vi "array2Mem_32bit_1to12_pipe.vi"(6 "Address (Max = 255)":u8=24, 10 "array_in":T1=[0.0, 0.0, 0.0, 0.0, 0.0, 0.0, 0.0, 0.0, 0.0, 0.0, 0.0, 0.0]) -> ()   [LabVIEW 2017]
uses:
  ziyi_pipe.ctl
  x_qp_scalar.ctl
  <vilib>/rvi/DataTransferAndStorage/Container/Common/niFpgaContainerExecOnDevCompGetState.vi
  <vilib>/rvi/Emulation/niFpgaEmulationIsFPGAContextNoSignature.vi
  <vilib>/rvi/DataTransferAndStorage/Container/Common/niFpgaContainerGetUniqueNameForEmu.vi
  <vilib>/rvi/Emulation/niFpgaProcessEmulError.vi
  <vilib>/rvi/Emulation/niFpgaSctlEmulationGetInTimedLoop.vi
  <vilib>/rvi/errors/nirviReportUnexpectedCaseInternalError (U32).vi
  <vilib>/rvi/Memory/Memory_Emulation/niFpgaMemoryEmulationCacheClearOnFirstRun.vi
  <vilib>/rvi/Memory/Memory_Emulation/nirvimemoryEmulationManagerCache_MakeExclusive.vi
  <vilib>/rvi/Memory/Memory_Emulation/niFpgaMemoryEmulationValidateCache.vi
  <vilib>/rvi/Memory/Memory_Emulation/nirvimemoryEmulationManagerCache_InsertValue.vi
  <vilib>/Utility/error.llb/Clear Errors.vi
  <vilib>/rvi/Memory/Memory_Emulation/nirvimemoryEmulationManagerCache_ReleaseExclusive.vi
  <vilib>/rvi/Memory/Memory_Emulation/nirvimemoryEmulationManagerCache_GetValue.vi
  <vilib>/rvi/Memory/Memory_Emulation/nirvimemoryEmulationManagerCache_SetValue.vi
  <vilib>/rvi/Emulation/niFpgaSctlEmulationResourceMgr.vi
  <vilib>/rvi/DataTransferAndStorage/Container/XNode/niFpgaContainer.xnode
  <vilib>/rvi/Memory/Memory_Emulation/niFpgaMemoryEmulationRefIn.vi
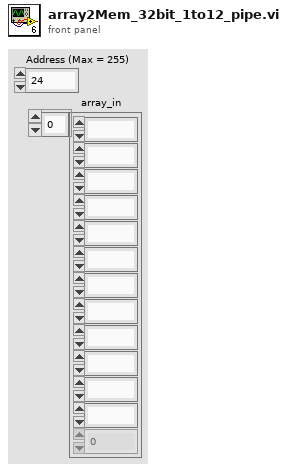
[diagram p1: front panel]
types:
  T1 = typedef "ziyi_pipe.ctl" = T2[]
  T2 = typedef "x_qp_scalar.ctl" = fxp<+/-,32,6>
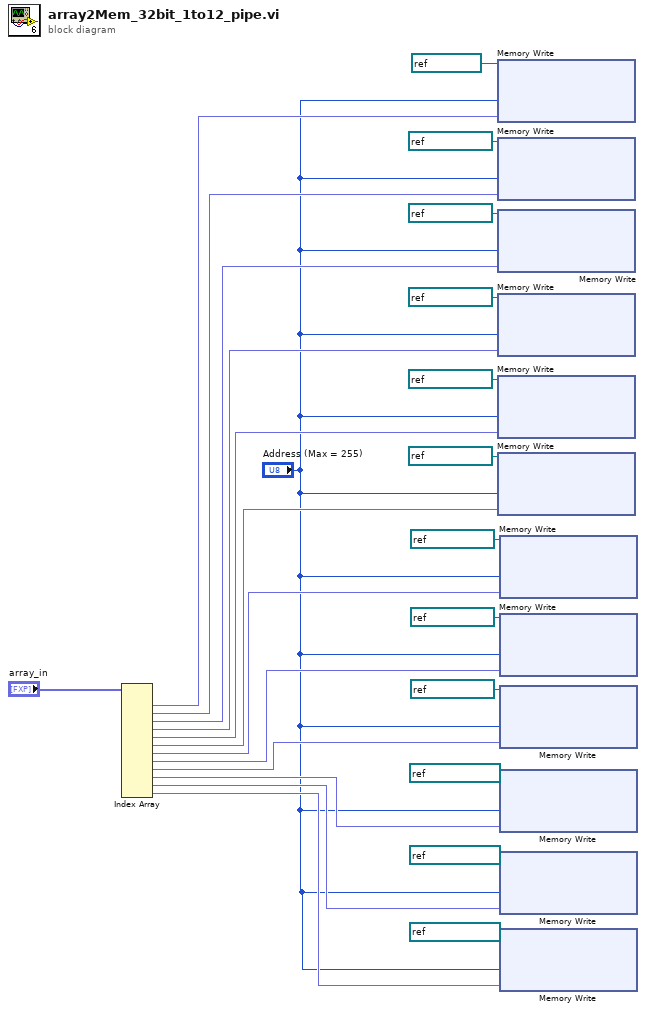
[diagram p0: block diagram]
diagram:
  n1 = Index Array(array="array_in") -> (element #1=w26:T2, element #2=w25:T2, element #3=w24:T2, element #4=w23:T2, element #5=w22:T2, element #6=w21:T2, element #7=w20:T2, element #8=w19:T2, element #9=w18:T2, element #10=w17:T2, element #11=w16:T2, element #12=w15:T2)  [unwired: 12 in]
  n2 = xnode ("Memory Write")("Address"="Address (Max = 255)", "Data"=w26, "Memory In"=refnum<k21> "Memory") -> ()  [unwired: 1 out]
  n3 = xnode ("Memory Write")("Address"="Address (Max = 255)", "Data"=w25, "Memory In"=refnum<k21> "Memory 2") -> ()  [unwired: 1 out]
  n4 = xnode ("Memory Write")("Address"="Address (Max = 255)", "Data"=w24, "Memory In"=refnum<k21> "Memory 3") -> ()  [unwired: 1 out]
  n5 = xnode ("Memory Write")("Address"="Address (Max = 255)", "Data"=w23, "Memory In"=refnum<k21> "Memory 4") -> ()  [unwired: 1 out]
  n6 = xnode ("Memory Write")("Address"="Address (Max = 255)", "Data"=w22, "Memory In"=refnum<k21> "Memory 5") -> ()  [unwired: 1 out]
  n7 = xnode ("Memory Write")("Address"="Address (Max = 255)", "Data"=w21, "Memory In"=refnum<k21> "Memory 6") -> ()  [unwired: 1 out]
  n8 = xnode ("Memory Write")("Address"="Address (Max = 255)", "Data"=w20, "Memory In"=refnum<k21> "Memory 7") -> ()  [unwired: 1 out]
  n9 = xnode ("Memory Write")("Address"="Address (Max = 255)", "Data"=w19, "Memory In"=refnum<k21> "Memory 8") -> ()  [unwired: 1 out]
  n10 = xnode ("Memory Write")("Address"="Address (Max = 255)", "Data"=w18, "Memory In"=refnum<k21> "Memory 9") -> ()  [unwired: 1 out]
  n11 = xnode ("Memory Write")("Address"="Address (Max = 255)", "Data"=w17, "Memory In"=refnum<k21> "Memory 10") -> ()  [unwired: 1 out]
  n12 = xnode ("Memory Write")("Address"="Address (Max = 255)", "Data"=w16, "Memory In"=refnum<k21> "Memory 11") -> ()  [unwired: 1 out]
  n13 = xnode ("Memory Write")("Address"="Address (Max = 255)", "Data"=w15, "Memory In"=refnum<k21> "Memory 12") -> ()  [unwired: 1 out]
